vi "Pockels-Adjust with Z.vi"(9 "Motor Z Planes(um)":dbl[](array[numeric])=[200.0, 150.0, 100.0, 50.0, 0.0, -50.0, -100.0, -150.0, -200.0]) -> (1 "Ls (Scattering Parameter)":dbl=100.0, 3 "Laser power % corrected for depth":dbl[](array[numeric]))   [LabVIEW 2017]
panel:
  in  "Disable AOL Z depth compensation":bool
  in  "Enable\nTest Input":bool
  in  "TEST INPUT":T1={"ZStack"={"Zstart"=200.0, "Zstop"=-200.0, "Zstep"=50.0}, "Laser Power %"={"@ Start"=10.0, "@ Stop"=80.0}}
  out "Waveform Graph":dbl[][](graph)
  out "Laser Power %.@ Stop":dbl
  out "Laser Power %.@ Start":dbl
  out "VI exec. time (ms)":u32
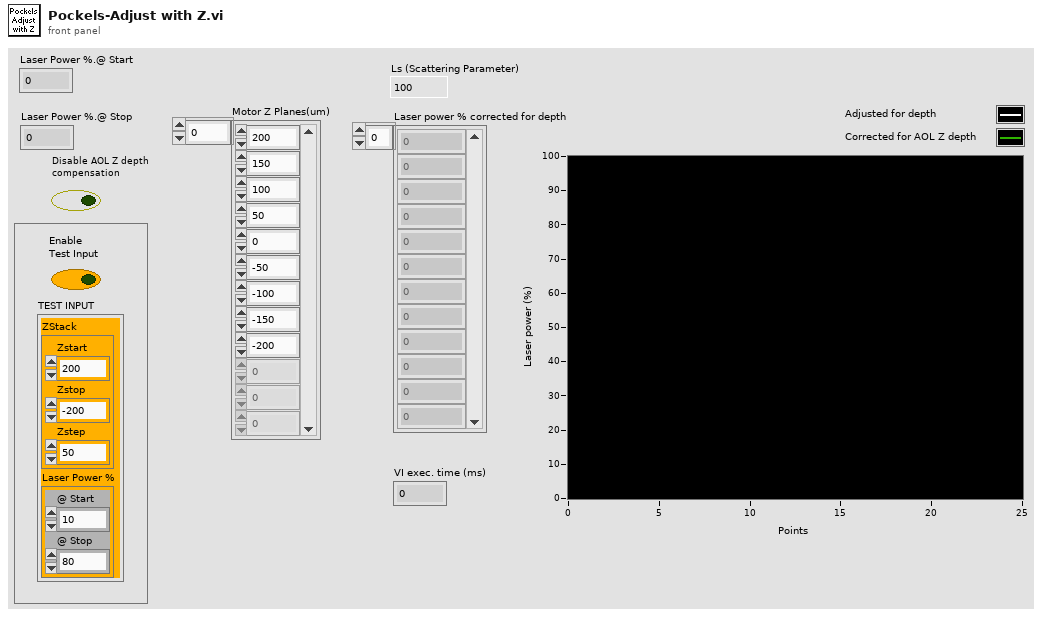
[diagram p1: front panel]
types:
  T1 = cluster{"ZStack":cluster{"Zstart":dbl, "Zstop":dbl, "Zstep":dbl}, "Laser Power %":cluster{"@ Start":dbl, "@ Stop":dbl}}
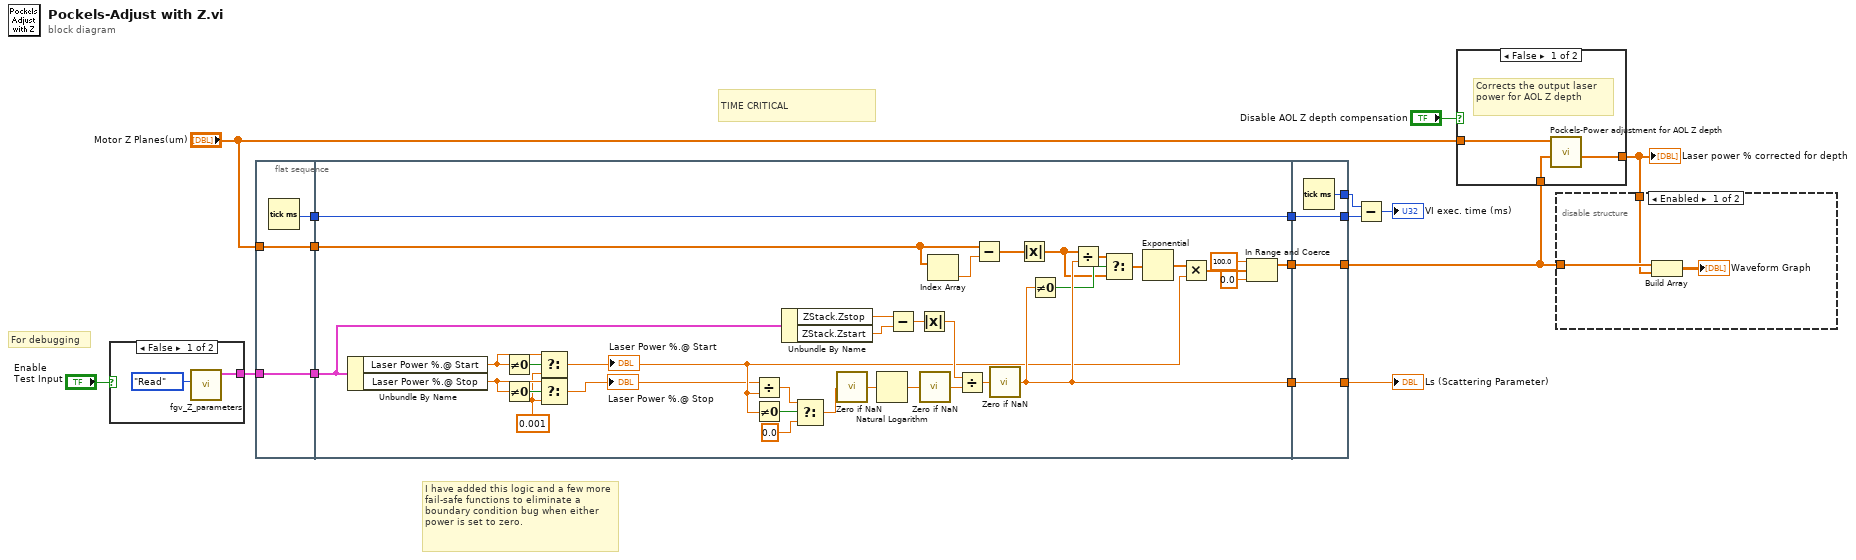
[diagram p0: block diagram]
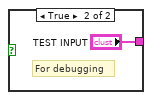
[diagram p4: hidden frame]
diagram:
  # "TIME CRITICAL"
  # "For debugging"
  # "I have added this logic and a few more fail-safe functions to eliminate a boundary condition bug when either power is set to zero."
  n1 = case shown="False" "Enable\nTest Input" {
    tunnel: [w18 "TEST INPUT"] -> w7
    frame False {
      n2 = call "fgv_Z_parameters.vi"("Function"=enum16{"Intialize", "Write", "Read", "Clear"}."Read") -> ("Z Parameters"=w18:T1)  [unwired: 9 in, 1 out]
    }
    frame True {
      # "For debugging"
    }
  }
  n3 = flat-sequence {
    tunnel: "Motor Z Planes(um)" -> [w21]
    tunnel: w7 -> [w22]
    tunnel: [w22] -> w14
    tunnel: [w21] -> w13
    tunnel: [w20] -> w11
    tunnel: [w47] -> w15
    tunnel: w14 -> [w39]
    tunnel: w13 -> [w53]
    tunnel: w11 -> [w51]
    tunnel: [w51] -> w10
    tunnel: [w23] -> w6
    tunnel: [w59] -> w16
    tunnel: [w60] -> w3
    tunnel: w15 -> [w59]
    tunnel: [w58] -> w12
    tunnel: w10 -> [w57]
    tunnel: [w57] -> w9
    tunnel: w6 -> [w60]
    frame #0 {
      n4 = Tick Count (ms)() -> (millisecond timer value=w20:u32)
    }
    frame #1 {
      w34 = 0.001 ("f")
      n5 = Unbundle By Name(w39) -> ("Laser Power %.@ Start"=w38:dbl, "Laser Power %.@ Stop"=w35:dbl)
      n6 = Not Equal To 0?(x=w38) -> (x != 0?=w40:bool)
      n7 = Not Equal To 0?(x=w35) -> (x != 0?=w36:bool)
      n8 = Select(t=w38, s=w40, f=w34) -> (s? t:f=w37:dbl)
      "Laser Power %.@ Start" <- w37
      n9 = Select(t=w35, s=w36, f=w34) -> (s? t:f=w33:dbl)
      "Laser Power %.@ Stop" <- w33
      n10 = Divide(x=w33, y=w37) -> (x/y=w32:dbl)
      n11 = Not Equal To 0?(x=w37) -> (x != 0?=w43:bool)
      n12 = Unbundle By Name(w39) -> ("ZStack.Zstop"=w41:dbl, "ZStack.Zstart"=w42:dbl)
      n13 = Select(t=w32, s=w43, f=0.0) -> (s? t:f=w30:dbl)
      n14 = call "Zero if NaN.vi"("Number In"=w30) -> ("Number Out"=w44:dbl)
      n15 = Natural Logarithm(1:w44) -> (0:w50:dbl)
      n16 = Subtract(x=w41, y=w42) -> (x-y=w55:dbl)
      n17 = Absolute Value(x=w55) -> (abs(x)=w56:dbl)
      n18 = call "Zero if NaN.vi"("Number In"=w50) -> ("Number Out"=w49:dbl)
      n19 = Index Array(array=w53) -> (element=w54:dbl)  [unwired: 1 in]
      n20 = Divide(x=w56, y=w49) -> (x/y=w48:dbl)
      n21 = Subtract(x=w53, y=w54) -> (x-y=w52:dbl[])
      n22 = call "Zero if NaN.vi"("Number In"=w48) -> ("Number Out"=w47:dbl)
      n23 = Absolute Value(x=w52) -> (abs(x)=w29:dbl[])
      n24 = Not Equal To 0?(x=w47) -> (x != 0?=w45:bool)
      n25 = Divide(x=w29, y=w47) -> (x/y=w28:dbl[])
      n26 = Select(t=w28, s=w45, f=w29) -> (s? t:f=w46:dbl[])
      n27 = Exponential(1:w46) -> (0:w27:dbl[])
      n28 = Multiply(x=w27, y=w37) -> (x*y=w24:dbl[])
      n29 = In Range and Coerce(upper limit=100.0, x=w24, lower limit=0.0) -> (coerced(x)=w23:dbl[])  [unwired: 1 out]
    }
    frame #2 {
      n30 = Tick Count (ms)() -> (millisecond timer value=w58:u32)
    }
  }
  n31 = Subtract(x=w12, y=w9) -> (x-y=→"VI exec. time (ms)":u32)
  n32 = case shown="False" "Disable AOL Z depth compensation" {
    tunnel: "Motor Z Planes(um)" -> [w63 _]
    tunnel: w3 -> [w62 w64]
    tunnel: [w61 w64] -> w2
    frame False {
      # "Corrects the output laser power for AOL Z depth"
      n33 = call "Pockels-Power adjustment for AOL Z depth.vi"("Laser power % corrected for depth"=w62, "Z planes um (xi)"=w63) -> ("Laser power % corrected for AOL Z depth"=w61:dbl[])  [unwired: 9 in]
    }
    frame True {
    }
  }
  "Laser power % corrected for depth" <- w2
  n34 = disable-structure shown="Enabled" {
    disable-tunnel: w3 -> [w66 _]
    disable-tunnel: w2 -> [w65 _]
    frame Enabled {
      n35 = Build Array(w66, w65) -> (→"Waveform Graph":dbl[][])
    }
    frame Disabled {
    }
  }
  "Ls (Scattering Parameter)" <- w16
